vi "ModbusCRCCalculator.vi"(1 "Input":u8[](array[numeric])) -> (0 "Output":u8[](array[numeric]))   [LabVIEW 2018, in "FPGAModbus.lvlib"]
uses:
  FPGAModbus.lvlib
panel:
  # "Calculates ModBus 16 bit CRC\n\nInput is array of uint8 values. Output is two\nuint8 values, representing CRC."
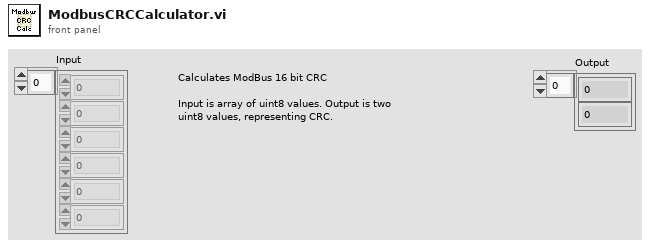
[diagram p1: front panel]
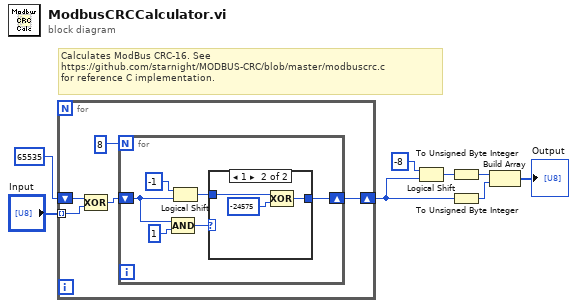
[diagram p0: block diagram]
diagram:
  # "Calculates ModBus CRC-16. See \nhttps://github.com/starnight/MODBUS-CRC/blob/master/modbuscrc.c\nfor reference C implementation."
  n1 = for {
    shift-right: [w9] -> w4
    shift-left: u16 65535 -> [w13]
    tunnel: "Input" -> [w12] mode=indexing
    n2 = Compound Arithmetic op=XOR(w13, w12) -> (w10:u16)
    n3 = for {
      N: i16 8 -> [_]
      shift-right: [w16] -> w9
      shift-left: w10 -> [w17]
      n4 = Logical Shift(y=i16 -1, x=w17) -> (x << y=w14:u16)
      n5 = Compound Arithmetic op=AND(w17, i16 1) -> (w19:u16)
      n6 = case shown="1" w19 {
        tunnel: [w20 w23] -> w16
        tunnel: w14 -> [w20 w21]
        frame 0, Default {
        }
        frame 1 {
          n7 = Compound Arithmetic op=XOR(w21, i16 -24575) -> (w23:u16)
        }
      }
    }
  }
  n8 = Logical Shift(y=i16 -8, x=w4) -> (x << y=w3:u16)
  n9 = To Unsigned Byte Integer(number=w3) -> (unsigned 8bit integer=w5:u8)
  n10 = To Unsigned Byte Integer(number=w4) -> (unsigned 8bit integer=w6:u8)
  n11 = Build Array(w5, w6) -> (→"Output":u8[])
